vi "Table.vi"(8 "Error In":errorcluster, 11 "Message Queues":T1) -> ()   [LabVIEW 2023, in "Weather Monitor Views.lvlib"]
doc: "Calls the Weather Monitor web service with different content-types and displays the raw data that is returned."
uses:
  Weather Monitor Views.lvlib
  support/Message Queue/All Message Queues.ctl
  support/Message Queue/Message Cluster.ctl
  Request/Response Data.ctl
  Application/Weather Data.ctl
  Application/Weather Data.lvlib
  support/Message Queue/Weather Message Queue.lvlib
  Weather Request Loop.lvlib
  support/User Event - Stop/Weather User Event - Stop.lvlib
panel:
  in  "Close button":bool
  out "Weather data":string[][](table)
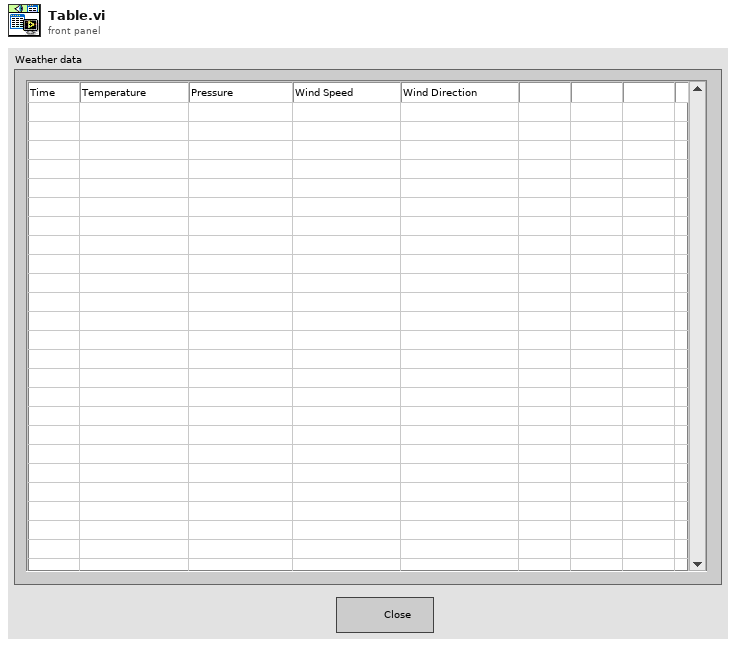
[diagram p1: front panel]
types:
  T1 = typedef "Weather Message Queue.lvlib/All Message Queues.ctl" = cluster{"View":refnum<queue>, "Request":refnum<queue>, "Wait":refnum<queue>}
  T2 = typedef "Weather Data.lvlib/Weather Data.ctl" = cluster{"Temperature":dbl, "Pressure":dbl, "Wind Speed":dbl, "Wind Direction":dbl}
  T3 = typedef "Weather Request Loop.lvlib/Response Data.ctl" = cluster{"Response Code":u16, "Body":string, "Headers":variant, "error":errorcluster}
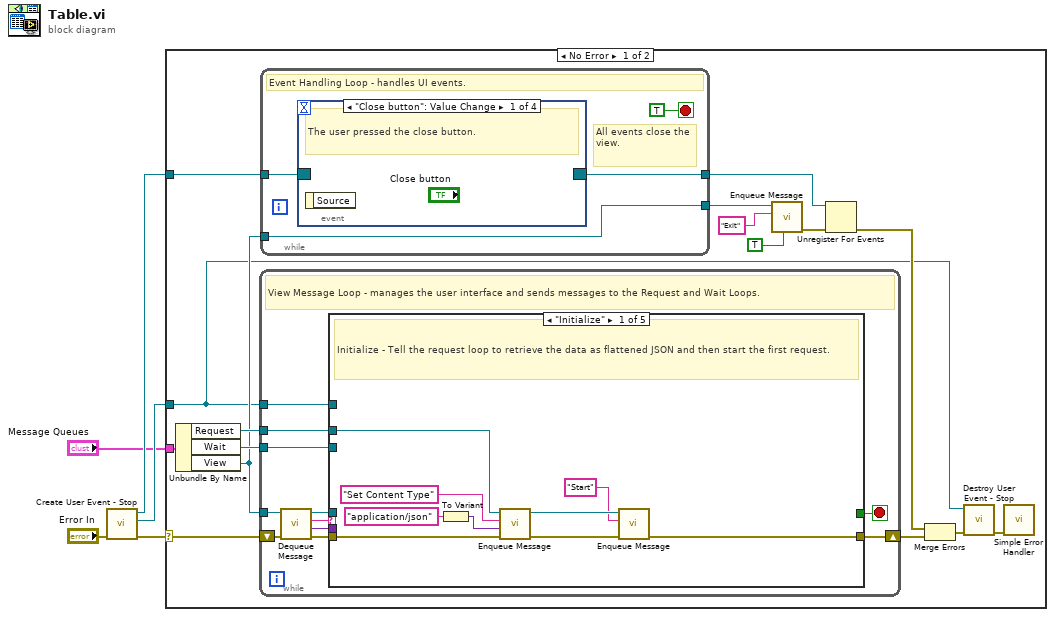
[diagram p0: block diagram]
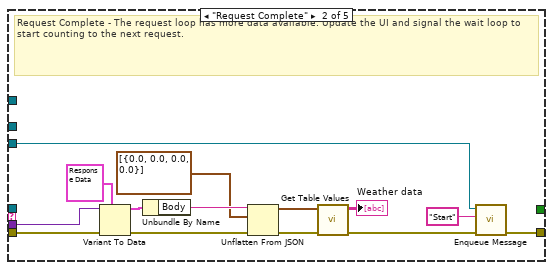
[diagram p2: hidden frame]
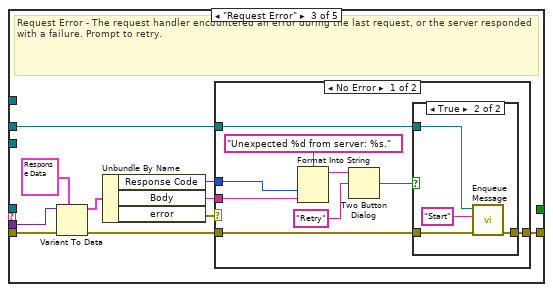
[diagram p3: hidden frame]
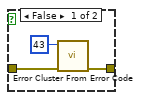
[diagram p4: hidden frame]
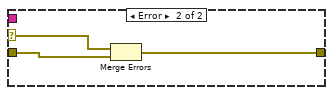
[diagram p5: hidden frame]
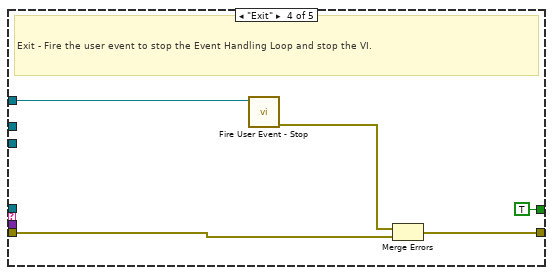
[diagram p6: hidden frame]
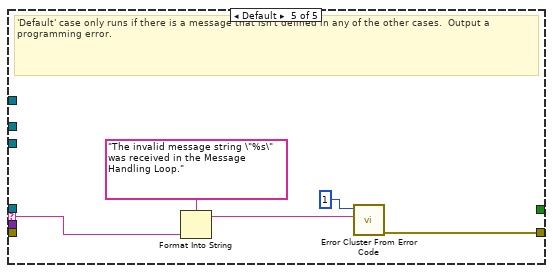
[diagram p7: hidden frame]
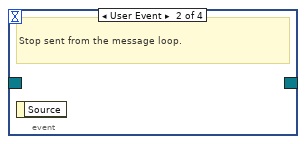
[diagram p8: hidden frame]
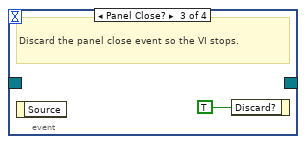
[diagram p9: hidden frame]
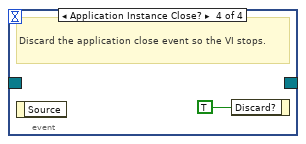
[diagram p10: hidden frame]
diagram:
  n1 = call "Create User Event - Stop.vi"("error in (no error)"="Error In") -> ("error out"=w5:errorcluster, "User Event - Stop"=w3:refnum<user-event>, "Stop Event Registration Refnum"=w4:refnum<event-registration>)  [unwired: 8 in]
  n2 = case shown="No Error" w5 {
    selector: w5 -> [w16 _]
    tunnel: "Message Queues" -> [w21 _]
    tunnel: w4 -> [w15 _]
    tunnel: w3 -> [w10 _]
    frame No Error {
      n3 = Unbundle By Name(w21) -> ("Request"=w20:refnum<queue>, "Wait"=w19:refnum<queue>, "View"=w18:refnum<queue>)
      n4 = while {
        tunnel: w20 -> [w24]
        tunnel: w19 -> [w25]
        tunnel: w18 -> [w32]
        shift-right: [w26] -> w17
        shift-left: w16 -> [w31]
        tunnel: w10 -> [w22]
        stop <- w23 stop-if-true
        # "View Message Loop - manages the user interface and sends messages to the Request and Wait Loops."
        n5 = call "Dequeue Message.vi"("error in (no error)"=w31, "Message Queue"=w32) -> ("error out"=w27:errorcluster, "Message Data"=w28:variant, "Message"=w30:string, "dup Message Queue"=w29:refnum<queue>)  [unwired: 6 in]
        n6 = case shown="\"Initialize\"" w30 {
          selector: w30 -> [_ _ _ _ w91]
          tunnel: w29 -> [_ _ _ _ _]
          tunnel: w28 -> [_ w54 w64 _ _]
          tunnel: w27 -> [w41 w55 w65 w85 _]
          tunnel: [w33 w51 w57 w86 w90] -> w26
          tunnel: w25 -> [_ w50 _ _ _]
          tunnel: w24 -> [w40 _ w56 _ _]
          tunnel: [_ _ _ TRUE _] -> w23
          tunnel: w22 -> [_ _ _ w88 _]
          frame "Initialize" {
            # "Initialize - Tell the request loop to retrieve the data as flattened JSON and then start the first request."
            n7 = To Variant(anything="application/json") -> (Variant=w37:variant)
            n8 = call "Enqueue Message.vi"("error in (no error)"=w41, "Message Data"=w37, "Message"="Set Content Type", "Message Queue"=w40) -> ("error out"=w35:errorcluster, "dup Message Queue"=w36:refnum<queue>)  [unwired: 6 in]
            n9 = call "Enqueue Message.vi"("error in (no error)"=w35, "Message"="Start", "Message Queue"=w36) -> ("error out"=w33:errorcluster)  [unwired: 7 in, 1 out]
          }
          frame "Request Complete" {
            # "Request Complete - The request loop has more data available. Update the UI and signal the wait loop to start counting to the next request."
            n10 = Variant To Data(error in=w55, type=T3 {"Response Code"=0, "Body"="", "Headers"=variant, "error"={"status"=FALSE, "code"=0, "source"=""}} ("Response Data"), Variant=w54) -> (data=w52:T3, error out=w45:errorcluster)
            n11 = Unbundle By Name(w52) -> ("Body"=w44:string)
            n12 = Unflatten From JSON(JSON string=w44, type and defaults=T2[] [{"Temperature"=0.0, "Pressure"=0.0, "Wind Speed"=0.0, "Wind Direction"=0.0}], error in (no error)=w45) -> (value=w48:T2[], error out=w47:errorcluster)  [unwired: 4 in]
            n13 = call "Get Table Values.vi"("error in (no error)"=w47, "Weather Data"=w48) -> ("error out"=w42:errorcluster, "Table Values"=→"Weather data":string[][])  [unwired: 8 in]
            n14 = call "Enqueue Message.vi"("error in (no error)"=w42, "Message"="Start", "Message Queue"=w50) -> ("error out"=w51:errorcluster)  [unwired: 7 in, 1 out]
          }
          frame "Request Error" {
            # "Request Error - The request handler encountered an error during the last request, or the server responded with a failure. Prompt to retry."
            n15 = Variant To Data(error in=w65, type=T3 {"Response Code"=0, "Body"="", "Headers"=variant, "error"={"status"=FALSE, "code"=0, "source"=""}} ("Response Data"), Variant=w64) -> (data=w62:T3, error out=w59:errorcluster)
            n16 = Unbundle By Name(w62) -> ("Response Code"=w61:u16, "Body"=w60:string, "error"=w58:errorcluster)
            n17 = case shown="No Error" w58 {
              selector: w58 -> [_ w84]
              tunnel: w61 -> [w71 _]
              tunnel: w60 -> [w70 _]
              tunnel: w59 -> [w69 w82]
              tunnel: [w68 w83] -> w57
              tunnel: w56 -> [w67 _]
              frame No Error {
                n18 = Format Into String(format string="Unexpected %d from server: %s.", w71, w70) -> (resulting string=w73:string)  [unwired: 2 in, 1 out]
                n19 = Two Button Dialog(message=w73, 2:"Retry" ("T button name (\"OK\")")) -> (T button?=w66:bool)  [unwired: 1 in]
                n20 = case shown="True" w66 {
                  tunnel: w69 -> [w76 w81]
                  tunnel: [w77 w80] -> w68
                  tunnel: w67 -> [_ w79]
                  frame False {
                    n21 = call <vilib>:"Error Cluster From Error Code.vi"("error in (no error)"=w76, "error code (0)"=43) -> ("error out"=w77:errorcluster)  [unwired: 7 in]
                  }
                  frame True {
                    n22 = call "Enqueue Message.vi"("error in (no error)"=w81, "Message"="Start", "Message Queue"=w79) -> ("error out"=w80:errorcluster)  [unwired: 7 in, 1 out]
                  }
                }
              }
              frame Error {
                n23 = Merge Errors(w84, w82) -> (w83:errorcluster)
              }
            }
          }
          frame "Exit" {
            # "Exit - Fire the user event to stop the Event Handling Loop and stop the VI."
            n24 = call "Fire User Event - Stop.vi"("User Event - Stop"=w88) -> ("error out"=w87:errorcluster)  [unwired: 10 in]
            n25 = Merge Errors(w87, w85) -> (w86:errorcluster)
          }
          frame Default {
            # "'Default' case only runs if there is a message that isn't defined in any of the other cases.  Output a programming error."
            n26 = Format Into String(format string="The invalid message string \"%s\" was received in the Message Handling Loop." ("Unknown Message Error Text"), w91) -> (resulting string=w92:string)  [unwired: 2 in, 1 out]
            n27 = call <vilib>:"Error Cluster From Error Code.vi"("error message (\"\")"=w92, "error code (0)"=1) -> ("error out"=w90:errorcluster)  [unwired: 7 in]
          }
        }
      }
      n28 = while {
        tunnel: w18 -> [w95]
        tunnel: w15 -> [w97]
        tunnel: [w96] -> w13
        tunnel: [w95] -> w6
        stop <- TRUE stop-if-true
        # "All events close the view."
        # "Event Handling Loop - handles UI events."
        n29 = event shown="[0] \"Close button\": Value Change" {
          selector: w97 -> [_ _ _ _]
          dyn-events: [_ _ _ _] -> w96
          timeout: _ -> [_ _ _ _]
          event "Close button": Value Change {
            # "The user pressed the close button."
            n30 = event-data() -> ()  [unwired: 1 in, 1 out]
          }
          event User Event {
            # "Stop sent from the message loop."
            n31 = event-data() -> ()  [unwired: 1 in, 1 out]
          }
          event Panel Close? {
            # "Discard the panel close event so the VI stops."
            n32 = event-data() -> ()  [unwired: 1 in, 1 out]
            n33 = event-data("Discard?"=TRUE) -> ()  [unwired: 1 in, 1 out]
          }
          event Application Instance Close? {
            # "Discard the application close event so the VI stops."
            n34 = event-data() -> ()  [unwired: 1 in, 1 out]
            n35 = event-data("Discard?"=TRUE) -> ()  [unwired: 1 in, 1 out]
          }
        }
      }
      n36 = call "Enqueue Message.vi"("Priority Message? (F)"=TRUE, "Message"="Exit", "Message Queue"=w6) -> ("error out"=w7:errorcluster)  [unwired: 7 in, 1 out]
      n37 = Unregister For Events(event registration refnum=w13, error in=w7) -> (error out=w14:errorcluster)
      n38 = Merge Errors(w14, w17) -> (w12:errorcluster)
      n39 = call "Destroy User Event - Stop.vi"("error in (no error)"=w12, "User Event - Stop"=w10) -> ("error out"=w11:errorcluster)  [unwired: 9 in]
      n40 = call <vilib>:"Simple Error Handler.vi"("error in (no error)"=w11) -> ()  [unwired: 4 in, 5 out]
    }
    frame Error {
    }
  }
